vi "Measurement Logic.vi"() -> ()   [LabVIEW 2021, in "NIDAQmxMeasurement.lvlib"]
uses:
  NIDAQmxMeasurement.lvlib
  <vilib>/Plug-In SDKs/Measurements/Measure Call Context/Measure Call Context.lvclass
  Measurement Configuration.ctl
  Measurement Results.ctl
  <vilib>/Plug-In SDKs/Measurements/Measure Call Context/Reserve Sessions - 1Pin.vi
  Source/Sessions/niDAQmx/Initialize Tasks - 1Task.vi
  <vilib>/Plug-In SDKs/Clients/Session Management V1/Session Reservation/Session Reservation.lvclass
  Source/Sessions/niDAQmx/Session Management niDAQmx.lvlib
panel:
  out "measurement results":T1
  in  "measurement configuration":T2
  out "measure call context out":refnum<class "Measure Call Context.lvclass">
  in  "measure call context in":refnum<class "Measure Call Context.lvclass">
  out "error out":errorcluster
  in  "error in":errorcluster
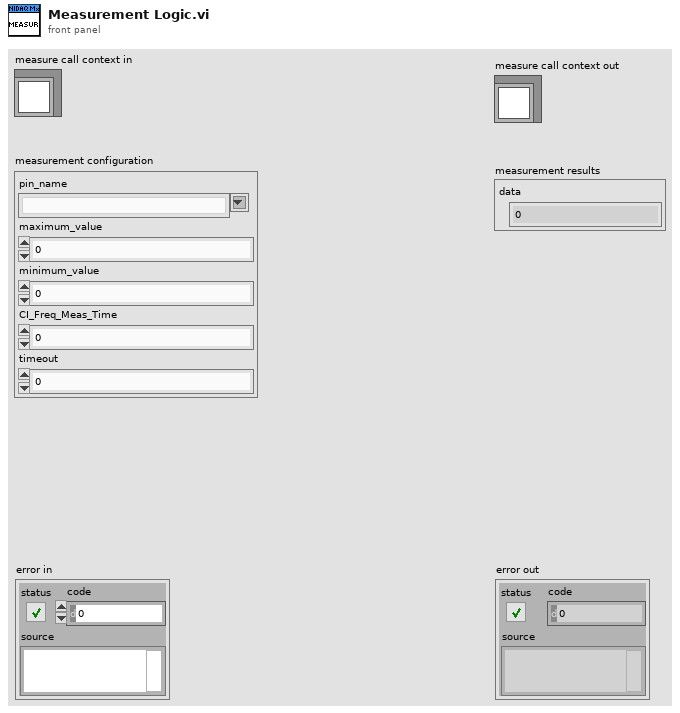
[diagram p1: front panel]
types:
  T1 = typedef "NIDAQmxMeasurement.lvlib/Measurement Results.ctl" = cluster{"data":dbl}
  T2 = typedef "NIDAQmxMeasurement.lvlib/Measurement Configuration.ctl" = cluster{"pin_name":string, "maximum_value":dbl, "minimum_value":dbl, "CI_Freq_Meas_Time":dbl, "timeout":dbl}
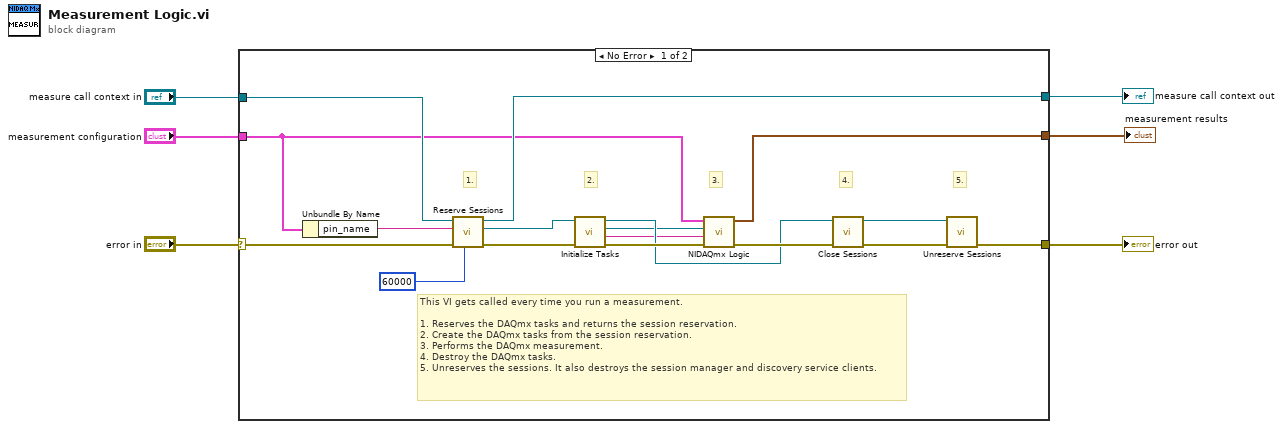
[diagram p0: block diagram]
diagram:
  n1 = case shown="No Error" "error in" {
    selector: "error in" -> [w21 w24]
    tunnel: "measure call context in" -> [w23 w25]
    tunnel: [w22 w25] -> w5
    tunnel: [w16 w24] -> w3
    tunnel: "measurement configuration" -> [w13 _]
    tunnel: [w14 _] -> w1
    frame No Error {
      # "2."
      # "This VI gets called every time you run a measurement.\n\n1. Reserves the DAQmx tasks and returns the session reservation.\n2. Create the DAQmx tasks from the session reservation. \n3. Performs the DAQmx measurement.\n4. Destroy the DAQmx tasks.\n5. Unreserves the sessions. It also destroys the session manager and discovery service clients."
      # "5."
      # "4."
      # "3."
      # "1."
      n2 = Unbundle By Name(w13) -> ("pin_name"=w9:string)
      n3 = call-poly <vilib>:"Reserve Sessions.vi"("timeout (ms)"=60000, "error in"=w21, "pin or relay name"=w9, "measurement context in"=w23) -> ("error out"=w11:errorcluster, "session reservation out"=w10:refnum<class "Session Reservation.lvclass">, "measurement context out"=w22:refnum<class "Measure Call Context.lvclass">)  [unwired: 5 in]
      n4 = call-poly "Initialize Tasks.vi"("error in"=w11, "session reservation in"=w10) -> ("error out"=w20:errorcluster, "channel list"=w8:string, "task"=w12:refnum<class "Session Factory.lvclass">, "session reservation out"=w18:refnum<class "Session Reservation.lvclass">)  [unwired: 6 in]
      n5 = call "NIDAQmx Logic.vi"("error in (no error)"=w20, "channel"=w8, "Session Factory in"=w12, "Measurement Configuration"=w13) -> ("error out"=w19:errorcluster, "Measurement Results"=w14:T1)  [unwired: 6 in]
      n6 = call <vilib>:"Close Sessions.vi"("error in"=w19, "session reservation in"=w18) -> ("error out"=w17:errorcluster, "session reservation out"=w15:refnum<class "Session Reservation.lvclass">)  [unwired: 8 in]
      n7 = call <vilib>:"Unreserve Sessions.vi"("error in"=w17, "session reservation in"=w15) -> ("error out"=w16:errorcluster)  [unwired: 9 in]
    }
    frame Error {
    }
  }
  "error out" <- w3
  "measure call context out" <- w5
  "measurement results" <- w1
